vi "DB Tools Select Data.vi"(4 "condition":string, 5 "error in (no error)":errorcluster, 6 "columns":string[](array[string]), 7 "table":string, 8 "connection reference":T1) -> (0 "error out":errorcluster, 1 "data":variant[][](array[variant]), 3 "connection reference out":T1)   [LabVIEW 2020, in "NI_Database_API.lvlib"]
doc: "Selects data from the <B>table</B> in the database identified by <B>connection reference</B> using the columns supplied in the <B>columns</B> array."
uses:
  <vilib>/addons/database/NI_Database_API.lvlib
  <vilib>/addons/database/Connection.llb/Conn ObjectReference.ctl
  <vilib>/addons/database/Connection.llb/Conn Execute.vi
  <vilib>/addons/database/Recordset.llb/Rec Fetch Recordset Data (R).vi
  <vilib>/addons/database/Recordset.llb/Rec Destroy - Connection.vi
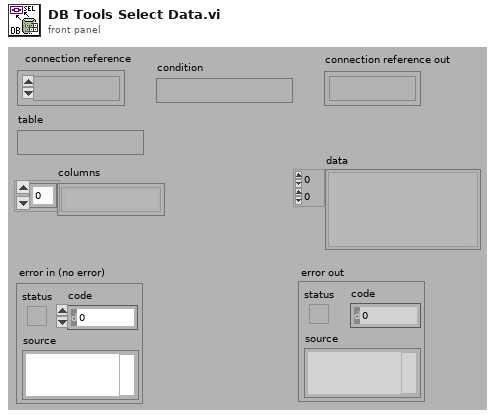
[diagram p1: front panel]
types:
  T1 = typedef "NI_Database_API.lvlib/Conn ObjectReference.ctl" = refnum<k1>
  T2 = typedef "NI_Database_API.lvlib/Rec ObjectReference.ctl" = refnum<k1>
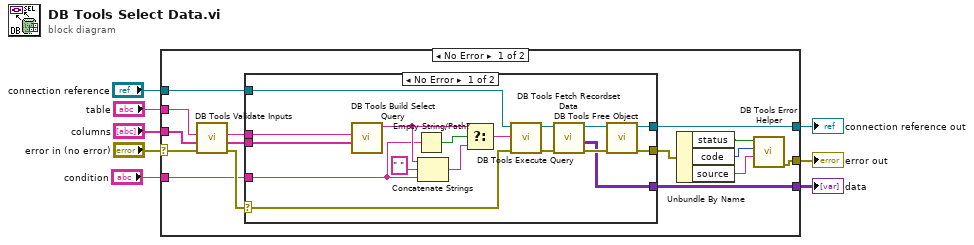
[diagram p0: block diagram]
diagram:
  n1 = case shown="No Error" "error in (no error)" {
    selector: "error in (no error)" -> [w9 w44]
    tunnel: "table" -> [w23 _]
    tunnel: [w15 w44] -> w7
    tunnel: "columns" -> [w14 _]
    tunnel: [w13 _] -> w5
    tunnel: [w12 w43] -> w4
    tunnel: "connection reference" -> [w11 w43]
    tunnel: "condition" -> [w10 _]
    frame No Error {
      n2 = call <vilib>:"DB Tools Validate Inputs.vi"("error in (no error)"=w9, "columns"=w14, "table"=w23) -> ("error out"=w19:errorcluster, "columns out"=w21:string[], "table out"=w20:string)  [unwired: 2 in]
      n3 = case shown="No Error" w19 {
        selector: w19 -> [w24 w42]
        tunnel: w21 -> [w25 _]
        tunnel: w20 -> [w40 _]
        tunnel: [w39 w42] -> w22
        tunnel: [w29 _] -> w13
        tunnel: [w28 w41] -> w12
        tunnel: w11 -> [w26 w41]
        tunnel: w10 -> [w27 _]
        frame No Error {
          n4 = call <vilib>:"DB Tools Build Select Query.vi"("columns"=w25, "table name"=w40) -> ("select query"=w33:string)  [unwired: 5 in]
          n5 = Empty String/Path?(string/path=w27) -> (empty?=w34:bool)
          n6 = Concatenate Strings(w33, " " ("Substring"), w27) -> (w32:string)
          n7 = Select(t=w33, s=w34, f=w32) -> (s? t:f=w30:string)
          n8 = call-poly <vilib>:"DB Tools Execute Query.vi"("error in (no error)"=w24, "SQL query"=w30, "connection reference"=w26) -> ("error out"=w36:errorcluster, "recordset reference"=w37:T2)  [unwired: 5 in]
          n9 = call-poly <vilib>:"DB Tools Fetch Recordset Data.vi"("error in (no error)"=w36, "recordset reference"=w37) -> ("error out"=w35:errorcluster, "recordset data"=w29:variant[][], "recordset reference out"=w38:T2)  [unwired: 3 in]
          n10 = call-poly <vilib>:"DB Tools Free Object.vi"("error in (no error)"=w35, "recordset reference"=w38) -> ("error out"=w39:errorcluster, "connection reference"=w28:T1)  [unwired: 8 in]
        }
        frame Error {
        }
      }
      n11 = Unbundle By Name(w22) -> ("status"=w18:bool, "code"=w17:i32, "source"=w16:string)
      n12 = call <vilib>:"DB Tools Error Helper.vi"("source"=w16, "code"=w17, "status"=w18) -> ("error out"=w15:errorcluster)  [unwired: 8 in]
    }
    frame Error {
    }
  }
  "error out" <- w7
  "data" <- w5
  "connection reference out" <- w4
